vi "Warnings.vi"(8 "error in (no error)":errorcluster, 9 "Минимальная":dbl, 10 "Максимальная":dbl, 11 "Текущая":dbl) -> (0 "error out":errorcluster, 1 "Предупреждение":bool, 2 "Текст":string)   [LabVIEW 2019]
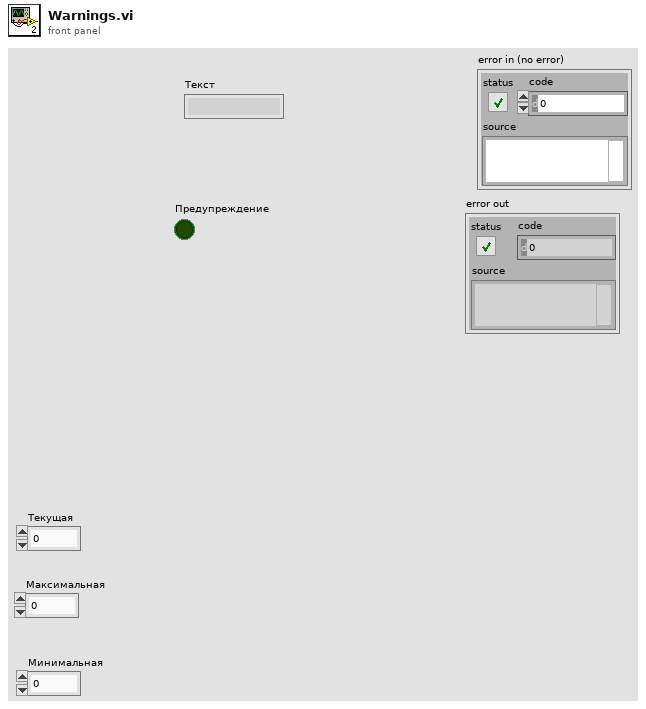
[diagram p1: front panel]
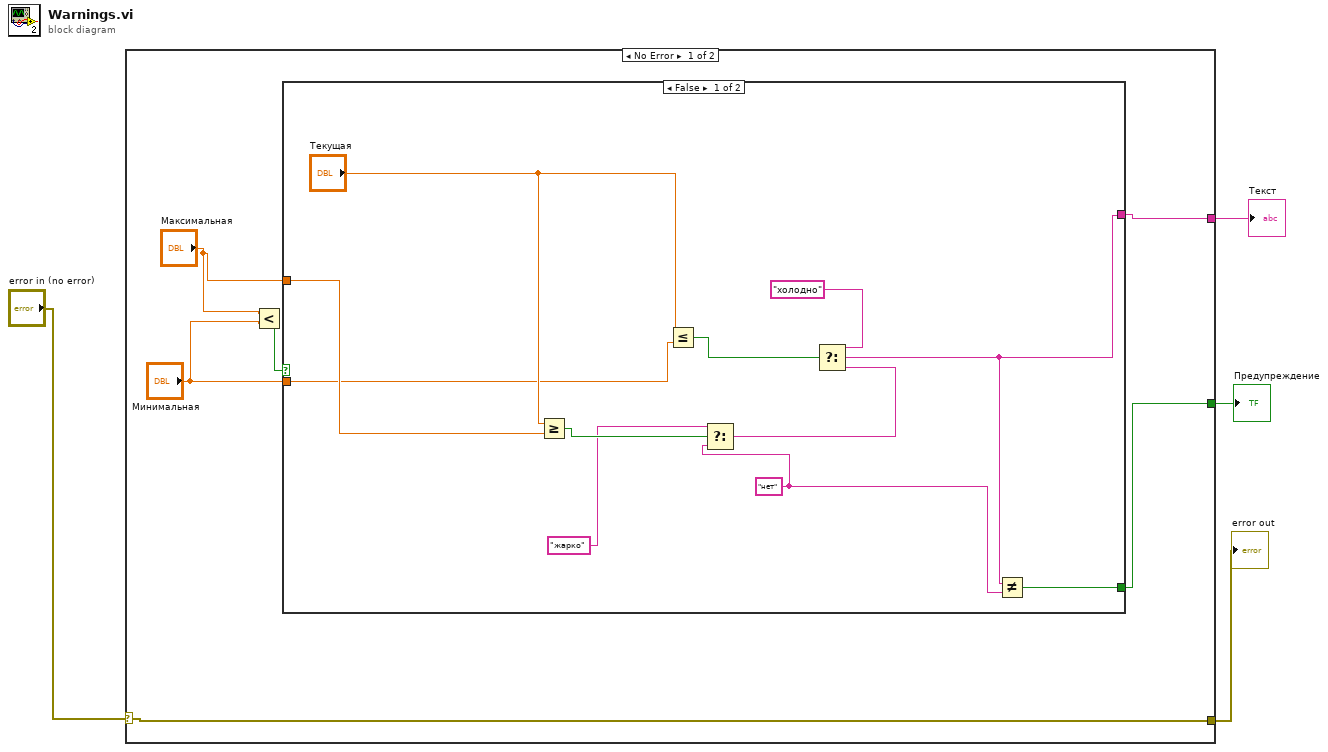
[diagram p0: block diagram]
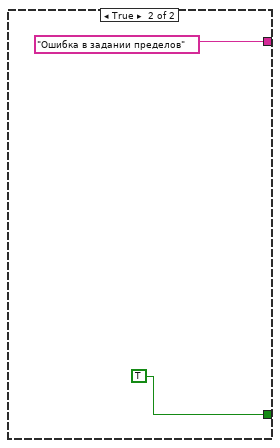
[diagram p2: hidden frame]
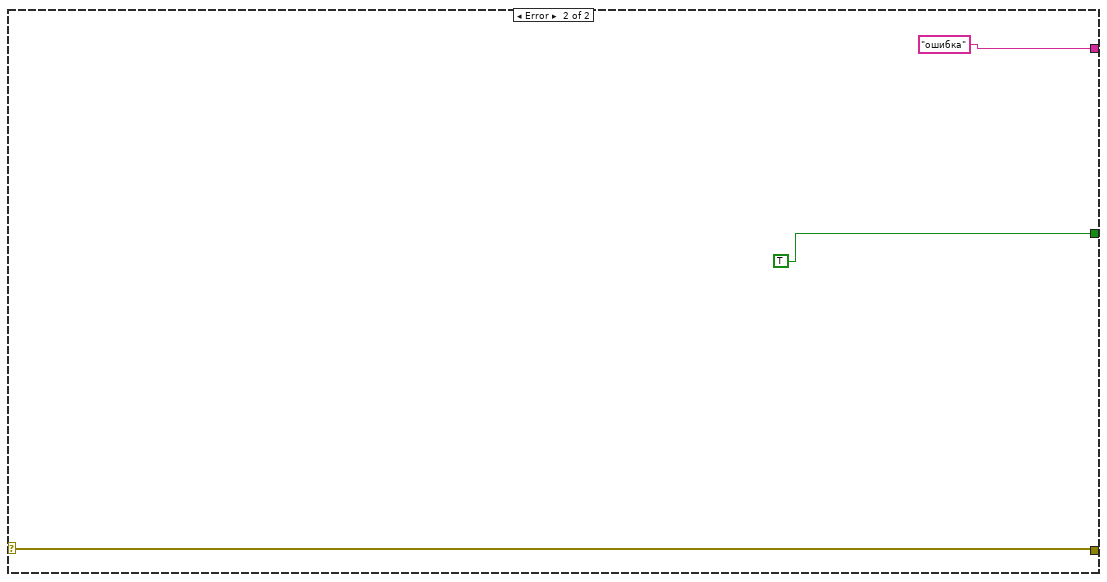
[diagram p3: hidden frame]
diagram:
  n1 = case shown="No Error" "error in (no error)" {
    selector: "error in (no error)" -> [w10 w25]
    tunnel: [w10 w25] -> w3
    tunnel: [w6 "ошибка"] -> w2
    tunnel: [w5 TRUE] -> w1
    frame No Error {
      n2 = Less?(x="Максимальная", y="Минимальная") -> (x < y?=w9:bool)
      n3 = case shown="False" w9 {
        tunnel: "Максимальная" -> [w14 _]
        tunnel: "Минимальная" -> [w13 _]
        tunnel: [w11 "Ошибка в задании пределов"] -> w6
        tunnel: [w12 TRUE] -> w5
        frame False {
          w18 = "нет"
          n4 = Greater Or Equal?(x="Текущая", y=w14) -> (x >= y?=w20:bool)
          n5 = Less Or Equal?(x="Текущая", y=w13) -> (x <= y?=w21:bool)
          n6 = Select(t="жарко", s=w20, f=w18) -> (s? t:f=w17:string)
          n7 = Select(t="холодно", s=w21, f=w17) -> (s? t:f=w11:string)
          n8 = Not Equal?(x=w11, y=w18) -> (x != y?=w12:bool)
        }
        frame True {
        }
      }
    }
    frame Error {
    }
  }
  "Текст" <- w2
  "Предупреждение" <- w1
  "error out" <- w3
